vi "Trim Whitespace 1.vi"   [LabVIEW 2009]
doc: "Removes leading and/or trailing whitespace from a string.\nWhitespace is defined as any of the following characters \\s \\t \\n \\0B \\f \\r.\nNon-printable is defined as any character less than ASCII 0x21.\n\nThis VI 's execution is set to <b>subroutine</b>\nThis VI is <b>reentrant</b>"
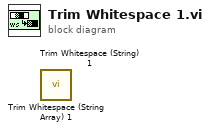
[diagram p0: block diagram]
diagram:
  n1 = call "Trim Whitespace (String Array) 1.vi"() -> ()  [unwired: 9 in, 1 out]
  n2 = call "Trim Whitespace (String) 1.vi"() -> ()  [unwired: 9 in, 1 out]
